vi "Ref Trig Buffer.vi"(0 "data in":u32, 1 "reset":bool, 5 "reference trigger":bool, 7 "pretrigger samples":u32, 9 "input valid":bool, 11 "abort":bool) -> (4 "data out":u32, 10 "output valid":bool, 13 "ready for reference":bool)   [LabVIEW 2014]
uses:
  Stream Buffer State.ctl
  <vilib>/rvi/DataTransferAndStorage/Container/Common/niFpgaContainerGetUniqueNameForEmu.vi
  <vilib>/rvi/DataTransferAndStorage/Container/Common/niFpgaContainerSetEmuInfo.vi
  <vilib>/rvi/eio/common/nirviEmuReportErrorAndStop.vi
  <vilib>/rvi/DataTransferAndStorage/Container/Common/niFpgaContainerExecOnDevCompGetState.vi
  <vilib>/rvi/Emulation/niFpgaEmulationIsFPGAContextNoSignature.vi
  <vilib>/rvi/Emulation/niFpgaProcessEmulError.vi
  <vilib>/rvi/Emulation/niFpgaSctlEmulationGetInTimedLoop.vi
  <vilib>/rvi/errors/nirviReportUnexpectedCaseInternalError (U32).vi
  <vilib>/rvi/Memory/Memory_Emulation/niFpgaMemoryEmulationCacheClearOnFirstRun.vi
  <vilib>/rvi/Memory/Memory_Emulation/nirvimemoryEmulationManagerCache_MakeExclusive.vi
  <vilib>/rvi/Memory/Memory_Emulation/niFpgaMemoryEmulationValidateCache.vi
  <vilib>/rvi/Memory/Memory_Emulation/nirvimemoryEmulationManagerCache_InsertValue.vi
  <vilib>/Utility/error.llb/Clear Errors.vi
  <vilib>/rvi/Memory/Memory_Emulation/nirvimemoryEmulationManagerCache_ReleaseExclusive.vi
  <vilib>/rvi/Memory/Memory_Emulation/nirvimemoryEmulationManagerCache_GetValue.vi
  <vilib>/rvi/Memory/Memory_Emulation/nirvimemoryEmulationManagerCache_SetValue.vi
  <vilib>/rvi/Emulation/niFpgaSctlEmulationResourceMgr.vi
  <vilib>/rvi/LocalResourceManager/LocalResourceManager.xnode
  <vilib>/rvi/DataTransferAndStorage/Container/XNode/niFpgaContainer.xnode
  <vilib>/rvi/Memory/Memory_Emulation/niFpgaMemoryEmulationRefIn.vi
  <vilib>/rvi/FXPMathLib/FxpInterpret/XNode/nifxpmath_Interpret.xnode
  <vilib>/rvi/FXPMathLib/FxpAdd/XNode/nifxpmath_Add.xnode
  <vilib>/rvi/FXPMathLib/sim/FxpSim.dll
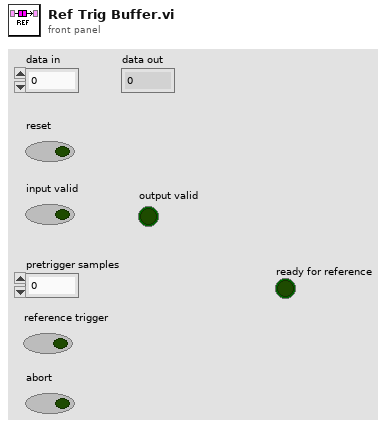
[diagram p1: front panel]
types:
  T1 = typedef "Stream Buffer State.ctl" = enum8{"Acquiring Pretrigger Samples", "Waiting for Reference Trigger", "Acquiring Posttrigger Samples"}
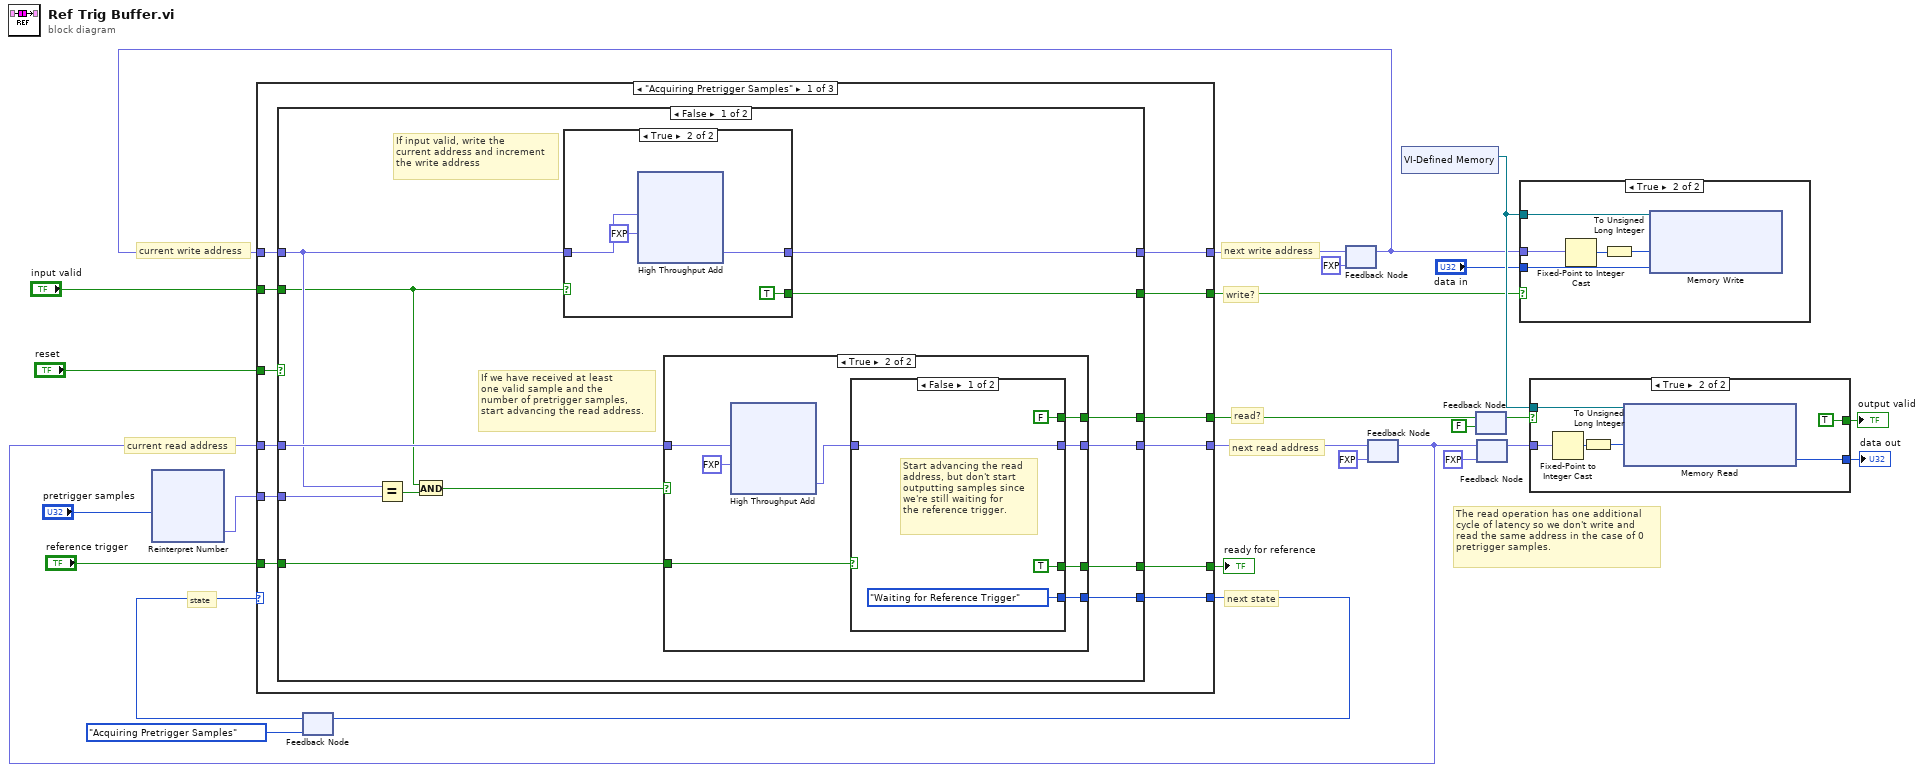
[diagram p0: block diagram]
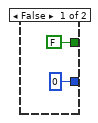
[diagram p2: hidden frame]
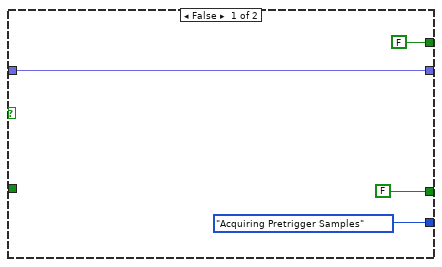
[diagram p4: hidden frame]
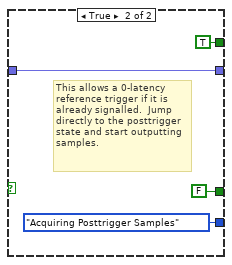
[diagram p5: hidden frame]
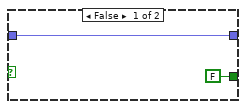
[diagram p6: hidden frame]
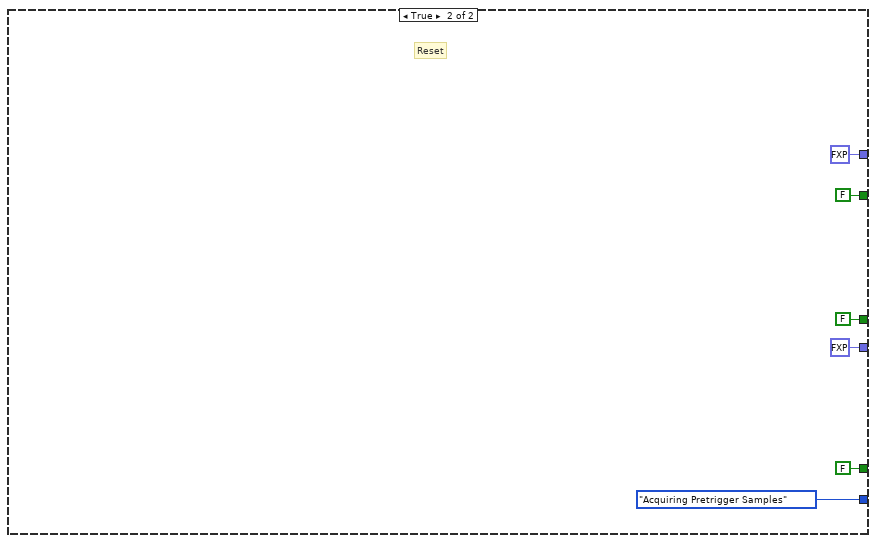
[diagram p7: hidden frame]
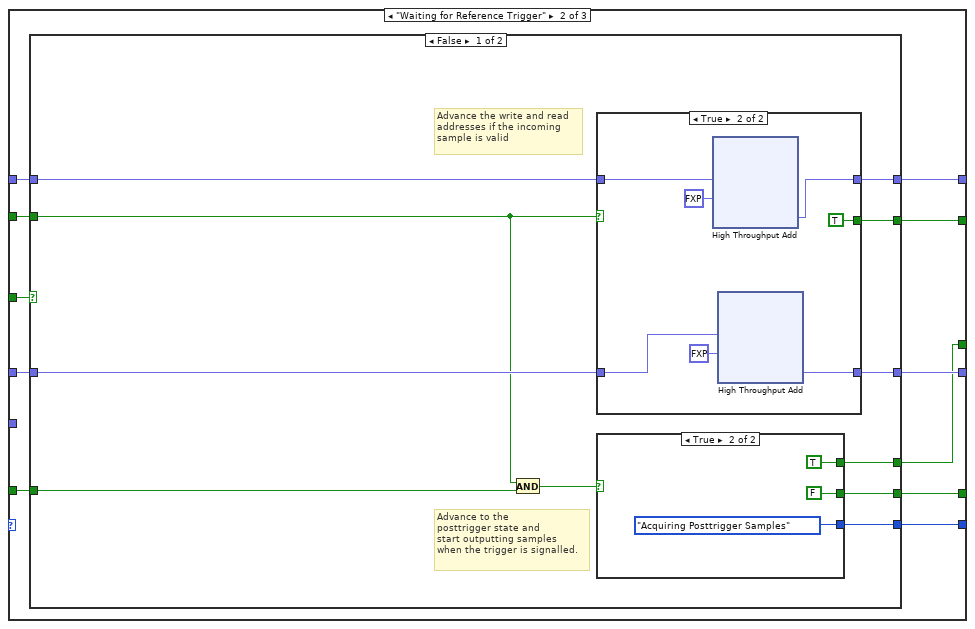
[diagram p8: hidden frame]
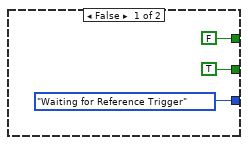
[diagram p9: hidden frame]
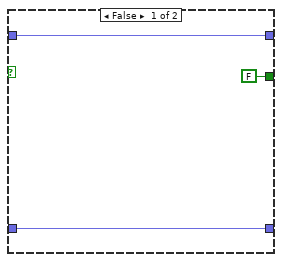
[diagram p10: hidden frame]
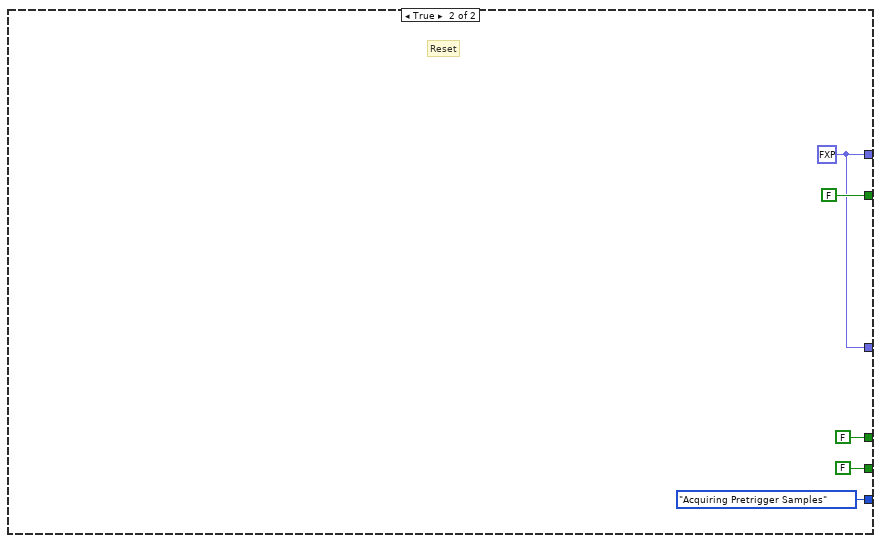
[diagram p11: hidden frame]
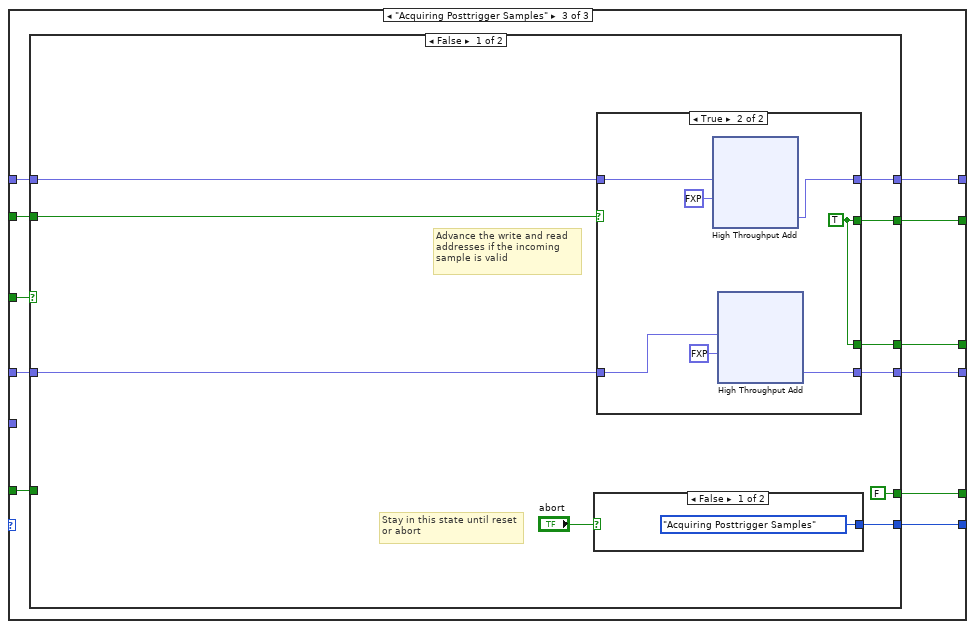
[diagram p12: hidden frame]
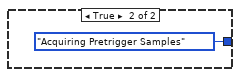
[diagram p13: hidden frame]
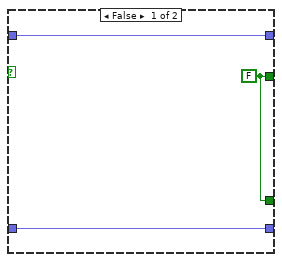
[diagram p14: hidden frame]
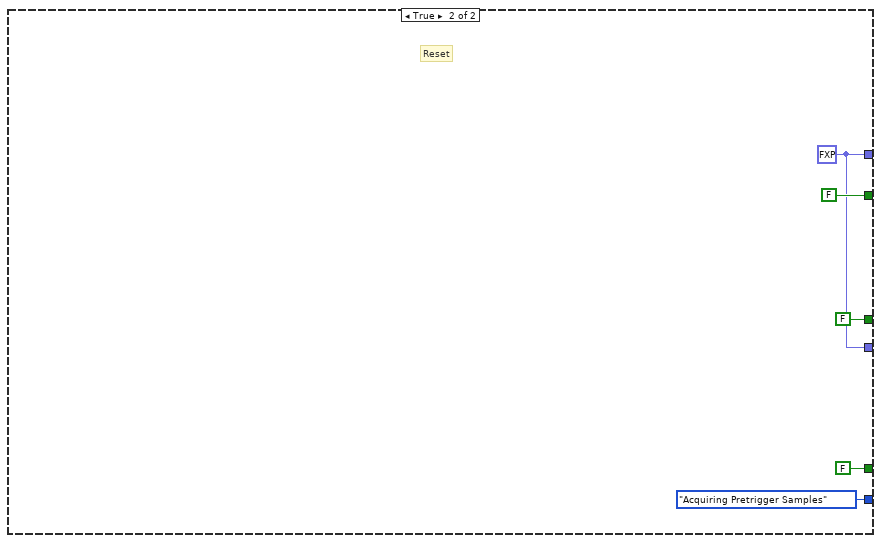
[diagram p15: hidden frame]
diagram:
  # "The read operation has one additional \ncycle of latency so we don't write and \nread the same address in the case of 0 \npretrigger samples."
  # "next state"
  # "state"
  # "current read address"
  # "current write address"
  # "next write address"
  # "next read address"
  # "read?"
  # "write?"
  n1 = xnode "Reinterpret Number"("x"="pretrigger samples") -> ("y"=w1:fxp<+,32,32>)
  n2 = feedback #1(Stream_Buffer_State."Acquiring Pretrigger Samples" ("Stream Buffer State")) -> (w24:T1)
  n3 = feedback #2(fxp<+,10,10> 0.0 ("y")) -> (w3:fxp<+,10,10>)
  n4 = feedback #3(fxp<+,10,10> 0.0 ("y")) -> (w5:fxp<+,10,10>)
  n5 = case shown="\"Acquiring Pretrigger Samples\"" w24 {
    tunnel: [w34 w90 w133] -> w22
    tunnel: [w26 w89 w132] -> w11
    tunnel: w5 -> [w31 w86 w129]
    tunnel: [w35 w91 w134] -> w21
    tunnel: [w28 w84 w126] -> w20
    tunnel: "input valid" -> [w33 w88 w131]
    tunnel: "reset" -> [w37 w93 w136]
    tunnel: [w36 w92 w135] -> w16
    tunnel: w3 -> [w30 w85 w128]
    tunnel: [w32 w87 w130] -> w15
    tunnel: "reference trigger" -> [w29 w83 w127]
    tunnel: w1 -> [w27 _ _]
    frame "Acquiring Pretrigger Samples" {
      n6 = case shown="False" w37 {
        tunnel: [w50 Stream_Buffer_State."Acquiring Pretrigger Samples" ("Stream Buffer State")] -> w36
        tunnel: [w41 FALSE] -> w35
        tunnel: [w44 fxp<+,10,10> 0.0 ("y")] -> w34
        tunnel: w33 -> [w39 _]
        tunnel: [w49 FALSE] -> w32
        tunnel: w31 -> [w48 _]
        tunnel: w30 -> [w40 _]
        tunnel: w29 -> [w47 _]
        tunnel: [w46 FALSE] -> w28
        tunnel: w27 -> [w45 _]
        tunnel: [w38 fxp<+,10,10> 0.0 ("y")] -> w26
        frame False {
          # "If we have received at least \none valid sample and the \nnumber of pretrigger samples,\nstart advancing the read address."
          # "If input valid, write the \ncurrent address and increment\nthe write address"
          n7 = Equal?(x=w40, y=w45) -> (x = y?=w42:bool)
          n8 = And(x=w39, y=w42) -> (x .and. y?=w43:bool)
          n9 = case shown="True" w39 {
            tunnel: [w71 w74] -> w44
            tunnel: [FALSE TRUE] -> w41
            tunnel: w40 -> [w71 w73]
            frame False {
            }
            frame True {
              n10 = xnode "High Throughput Add"("x"=w73, "y"=fxp<+,10,10> 1.0) -> ("x+y"=w74:fxp<+,10,10>)
            }
          }
          n11 = case shown="True" w43 {
            tunnel: [Stream_Buffer_State."Acquiring Pretrigger Samples" ("Stream Buffer State") w62] -> w50
            tunnel: [FALSE w61] -> w49
            tunnel: w48 -> [w51 w56]
            tunnel: w47 -> [_ w60]
            tunnel: [FALSE w59] -> w46
            tunnel: [w51 w58] -> w38
            frame False {
            }
            frame True {
              n12 = xnode "High Throughput Add"("x"=w56, "y"=fxp<+,10,10> 1.0) -> ("x+y"=w55:fxp<+,10,10>)
              n13 = case shown="False" w60 {
                tunnel: [Stream_Buffer_State."Waiting for Reference Trigger" ("Stream Buffer State") Stream_Buffer_State."Acquiring Posttrigger Samples" ("Stream Buffer State")] -> w62
                tunnel: [TRUE FALSE] -> w61
                tunnel: [FALSE TRUE] -> w59
                tunnel: [w63 w67] -> w58
                tunnel: w55 -> [w63 w67]
                frame False {
                  # "Start advancing the read\naddress, but don't start\noutputting samples since\nwe're still waiting for \nthe reference trigger."
                }
                frame True {
                  # "This allows a 0-latency\nreference trigger if it is\nalready signalled.  Jump\ndirectly to the posttrigger\nstate and start outputting\nsamples."
                }
              }
            }
          }
        }
        frame True {
          # "Reset"
        }
      }
    }
    frame "Waiting for Reference Trigger" {
      n14 = case shown="False" w93 {
        tunnel: [w102 Stream_Buffer_State."Acquiring Pretrigger Samples" ("Stream Buffer State")] -> w92
        tunnel: [w103 FALSE] -> w91
        tunnel: [w104 w121] -> w90
        tunnel: [w99 w121] -> w89
        tunnel: w88 -> [w94 _]
        tunnel: [w101 FALSE] -> w87
        tunnel: w86 -> [w98 _]
        tunnel: w85 -> [w100 _]
        tunnel: [w97 FALSE] -> w84
        tunnel: w83 -> [w96 _]
        frame False {
          # "Advance to the \nposttrigger state and \nstart outputting samples\nwhen the trigger is signalled."
          # "Advance the write and read\naddresses if the incoming\nsample is valid"
          n15 = And(x=w94, y=w96) -> (x .and. y?=w95:bool)
          n16 = case shown="True" w94 {
            tunnel: [w113 w117] -> w104
            tunnel: [FALSE TRUE] -> w103
            tunnel: w100 -> [w113 w118]
            tunnel: [w111 w114] -> w99
            tunnel: w98 -> [w111 w115]
            frame False {
            }
            frame True {
              n17 = xnode "High Throughput Add"("x"=w118, "y"=fxp<+,10,10> 1.0) -> ("x+y"=w117:fxp<+,10,10>)
              n18 = xnode "High Throughput Add"("x"=w115, "y"=fxp<+,10,10> 1.0) -> ("x+y"=w114:fxp<+,10,10>)
            }
          }
          n19 = case shown="True" w95 {
            tunnel: [Stream_Buffer_State."Waiting for Reference Trigger" ("Stream Buffer State") Stream_Buffer_State."Acquiring Posttrigger Samples" ("Stream Buffer State")] -> w102
            tunnel: [TRUE FALSE] -> w101
            tunnel: [FALSE TRUE] -> w97
            frame False {
            }
            frame True {
            }
          }
        }
        frame True {
          w121 = fxp<+,10,10> 0.0 ("y")
          # "Reset"
        }
      }
    }
    frame "Acquiring Posttrigger Samples" {
      n20 = case shown="False" w136 {
        tunnel: [w144 Stream_Buffer_State."Acquiring Pretrigger Samples" ("Stream Buffer State")] -> w135
        tunnel: [w145 FALSE] -> w134
        tunnel: [w146 w160] -> w133
        tunnel: [w141 w160] -> w132
        tunnel: w131 -> [w139 _]
        tunnel: [FALSE FALSE] -> w130
        tunnel: w129 -> [w140 _]
        tunnel: w128 -> [w142 _]
        tunnel: w127 -> [_ _]
        tunnel: [w138 FALSE] -> w126
        frame False {
          # "Stay in this state until reset\nor abort"
          # "Advance the write and read\naddresses if the incoming\nsample is valid"
          n21 = case shown="False" "abort" {
            tunnel: [Stream_Buffer_State."Acquiring Posttrigger Samples" ("Stream Buffer State") Stream_Buffer_State."Acquiring Pretrigger Samples" ("Stream Buffer State")] -> w144
            frame False {
            }
            frame True {
            }
          }
          n22 = case shown="True" w139 {
            tunnel: [w151 w156] -> w146
            tunnel: [w149 w152] -> w145
            tunnel: w142 -> [w151 w157]
            tunnel: [w150 w153] -> w141
            tunnel: w140 -> [w150 w154]
            tunnel: [w149 w152] -> w138
            frame False {
              w149 = FALSE
            }
            frame True {
              w152 = TRUE
              n23 = xnode "High Throughput Add"("x"=w157, "y"=fxp<+,10,10> 1.0) -> ("x+y"=w156:fxp<+,10,10>)
              n24 = xnode "High Throughput Add"("x"=w154, "y"=fxp<+,10,10> 1.0) -> ("x+y"=w153:fxp<+,10,10>)
            }
          }
        }
        frame True {
          w160 = fxp<+,10,10> 0.0 ("y")
          # "Reset"
        }
      }
    }
  }
  "ready for reference" <- w15
  n25 = feedback-in #1(w16) -> ()
  n26 = feedback-in #2(w22) -> ()
  n27 = feedback-in #3(w11) -> ()
  n28 = xnode "VI-Defined Memory"() -> ("Memory Out"=w23:refnum<k21>)
  n29 = feedback-in #4(w20) -> ()
  n30 = feedback #4(FALSE) -> (w10:bool)
  n31 = feedback #5(fxp<+,10,10> 0.0 ("y")) -> (w4:fxp<+,10,10>)
  n32 = feedback-in #5(w5) -> ()
  n33 = case shown="True" w21 {
    tunnel: w23 -> [_ w168]
    tunnel: w3 -> [_ w166]
    tunnel: "data in" -> [_ w167]
    frame False {
    }
    frame True {
      n34 = Fixed-Point to Integer Cast(1:w166) -> (0:w165:u16)
      n35 = To Unsigned Long Integer(number=w165) -> (unsigned 32bit integer=w164:u32)
      n36 = xnode "Memory Write"("Address"=w164, "Data"=w167, "Memory In"=w168) -> ()  [unwired: 1 out]
    }
  }
  n37 = case shown="True" w10 {
    tunnel: w23 -> [_ w176]
    tunnel: [u32 0 ("Data") w175] -> w14
    tunnel: [FALSE TRUE] -> w13
    tunnel: w4 -> [_ w172]
    frame False {
    }
    frame True {
      n38 = Fixed-Point to Integer Cast(1:w172) -> (0:w173:u16)
      n39 = To Unsigned Long Integer(number=w173) -> (unsigned 32bit integer=w171:u32)
      n40 = xnode "Memory Read"("Address"=w171, "Memory In"=w176) -> ("Data"=w175:u32)  [unwired: 1 out]
    }
  }
  "output valid" <- w13
  "data out" <- w14
